vi "FPGA_FTL_trigger_camera_synchro_laser_lines.vi"(3 "N Z positions":i32) -> ()   [LabVIEW 2015]
uses:
  <vilib>/Platform/TimedLoop/XDataNode/timing_clust.ctl
  <vilib>/Platform/TimedLoop/XDataNode/nitl_modes.ctl
  <vilib>/Platform/TimedLoop/XDataNode/wakeup.ctl
  <vilib>/rvi/FXPMathLib/basic elements/FxpIntAccumulator/subVIs/nifxpmath_IntAccumulator_SimConfig.ctl
  <vilib>/rvi/Emulation/niFpgaGetClockAttributes.vi
  <vilib>/rvi/Emulation/niFpgaSctlEmulationGetInTimedLoop.vi
  <vilib>/rvi/Emulation/niFpgaEmulationReportErrorSimple.vi
  <vilib>/rvi/eio/common/nirviEmuTemplateMethod_errors.vi
  <vilib>/rvi/Emulation/niFpgaCriticalErrorInLSC.vi
  <vilib>/rvi/Emulation/niFpgaProcessEmulError.vi
  <vilib>/rvi/Analysis/common/codeGenErrors/XNode/niFpgaXNodeCodeGenErrorHandle.vi
  <vilib>/rvi/FXPMathLib/basic elements/FxpIntAccumulator/simVIs/DllFxpIntAccumulator_sub.vi
  <vilib>/eio/EIONode/EIONode.xnode
  <vilib>/rvi/Analysis/measure/dc-rms/XNode/niFpgaDC-RMS.xnode
  <vilib>/Platform/TimedLoop/XDataNode/XDataNode.xnode
  <vilib>/rvi/FXPMathLib/basic elements/FxpIntAccumulator/XNode/nifxpmath_IntAccumulator.xnode
  <vilib>/Platform/TimedLoop/XDataNode/XDNodeRunTimeDep.lvlib
panel:
  in  "stop":bool
  out "duration (ms)":u32
  out "QPD":T1
  in  "Reset counter":bool
  in  "Count(uSec)":u32=100
  out "Images acquired":i32
  in  "Laser lines":i32[](array[numeric])=[0, 0, 0, 0, 0]
  in  "Laser power":sgl[](array[numeric])=[0.0, 0.0, 0.0, 0.0, 0.0]
  in  "N laser lines":i32
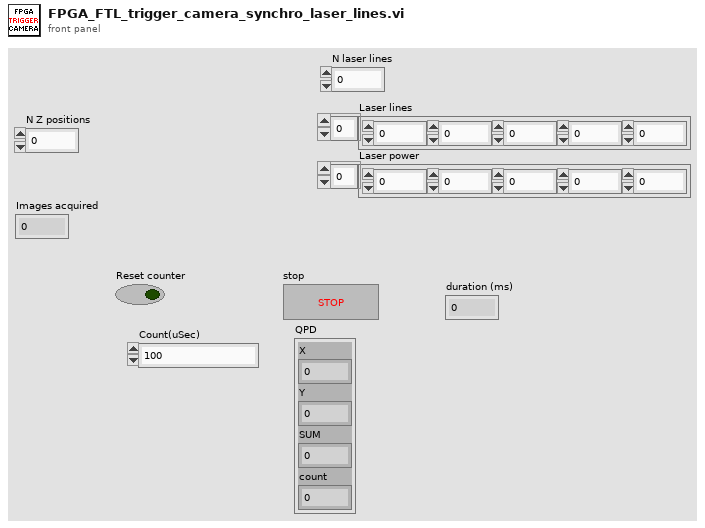
[diagram p1: front panel]
types:
  T1 = cluster{"X":sgl, "Y":sgl, "SUM":sgl, "count":u32}
  T2 = typedef "XDNodeRunTimeDep.lvlib/timing_clust.ctl" = cluster{"Expected End [f-1]":u64, "Actual End [f-1]":u64, "Finished Late? [f-1]":bool, "Expected End [i-1]":u64, "Actual End [i-1]":u64, "Finished Late? [i-1]":bool, "Expected Start [i]":u64, "Actual Start [i]":u64, "Expected Start [f]":u64, "Actual Start [f]":u64, "Source Name":string, "Structure Name":string, "Period":i64, "Deadline":i64, "Offset":i64, "Start":i64, "Priority":i32, "Timeout":i32, "Mode":T3, "Wakeup Reason":T4, "Error":errorcluster, "Source Type":string, "Secondary Source Type":string, "Global End Time":u64, "Global Start Time":u64, "Frame Duration":u64, "Iteration Duration":u64, "Assigned CPU":i32, "I/O Scan Engine Mode":u32}
  T3 = typedef "XDNodeRunTimeDep.lvlib/nitl_modes.ctl" = enum32{"No Change", "Process missed periods, maintain original phase", "Discard missed periods, maintain original phase", "Process missed periods, ignore original phase", "Discard missed periods, ignore original phase"}
  T4 = typedef "XDNodeRunTimeDep.lvlib/wakeup.ctl" = enum32{"Normal", "Aborted", "Asynchronous wakeup", "Timing source error", "Timed loop error", "Timeout"}
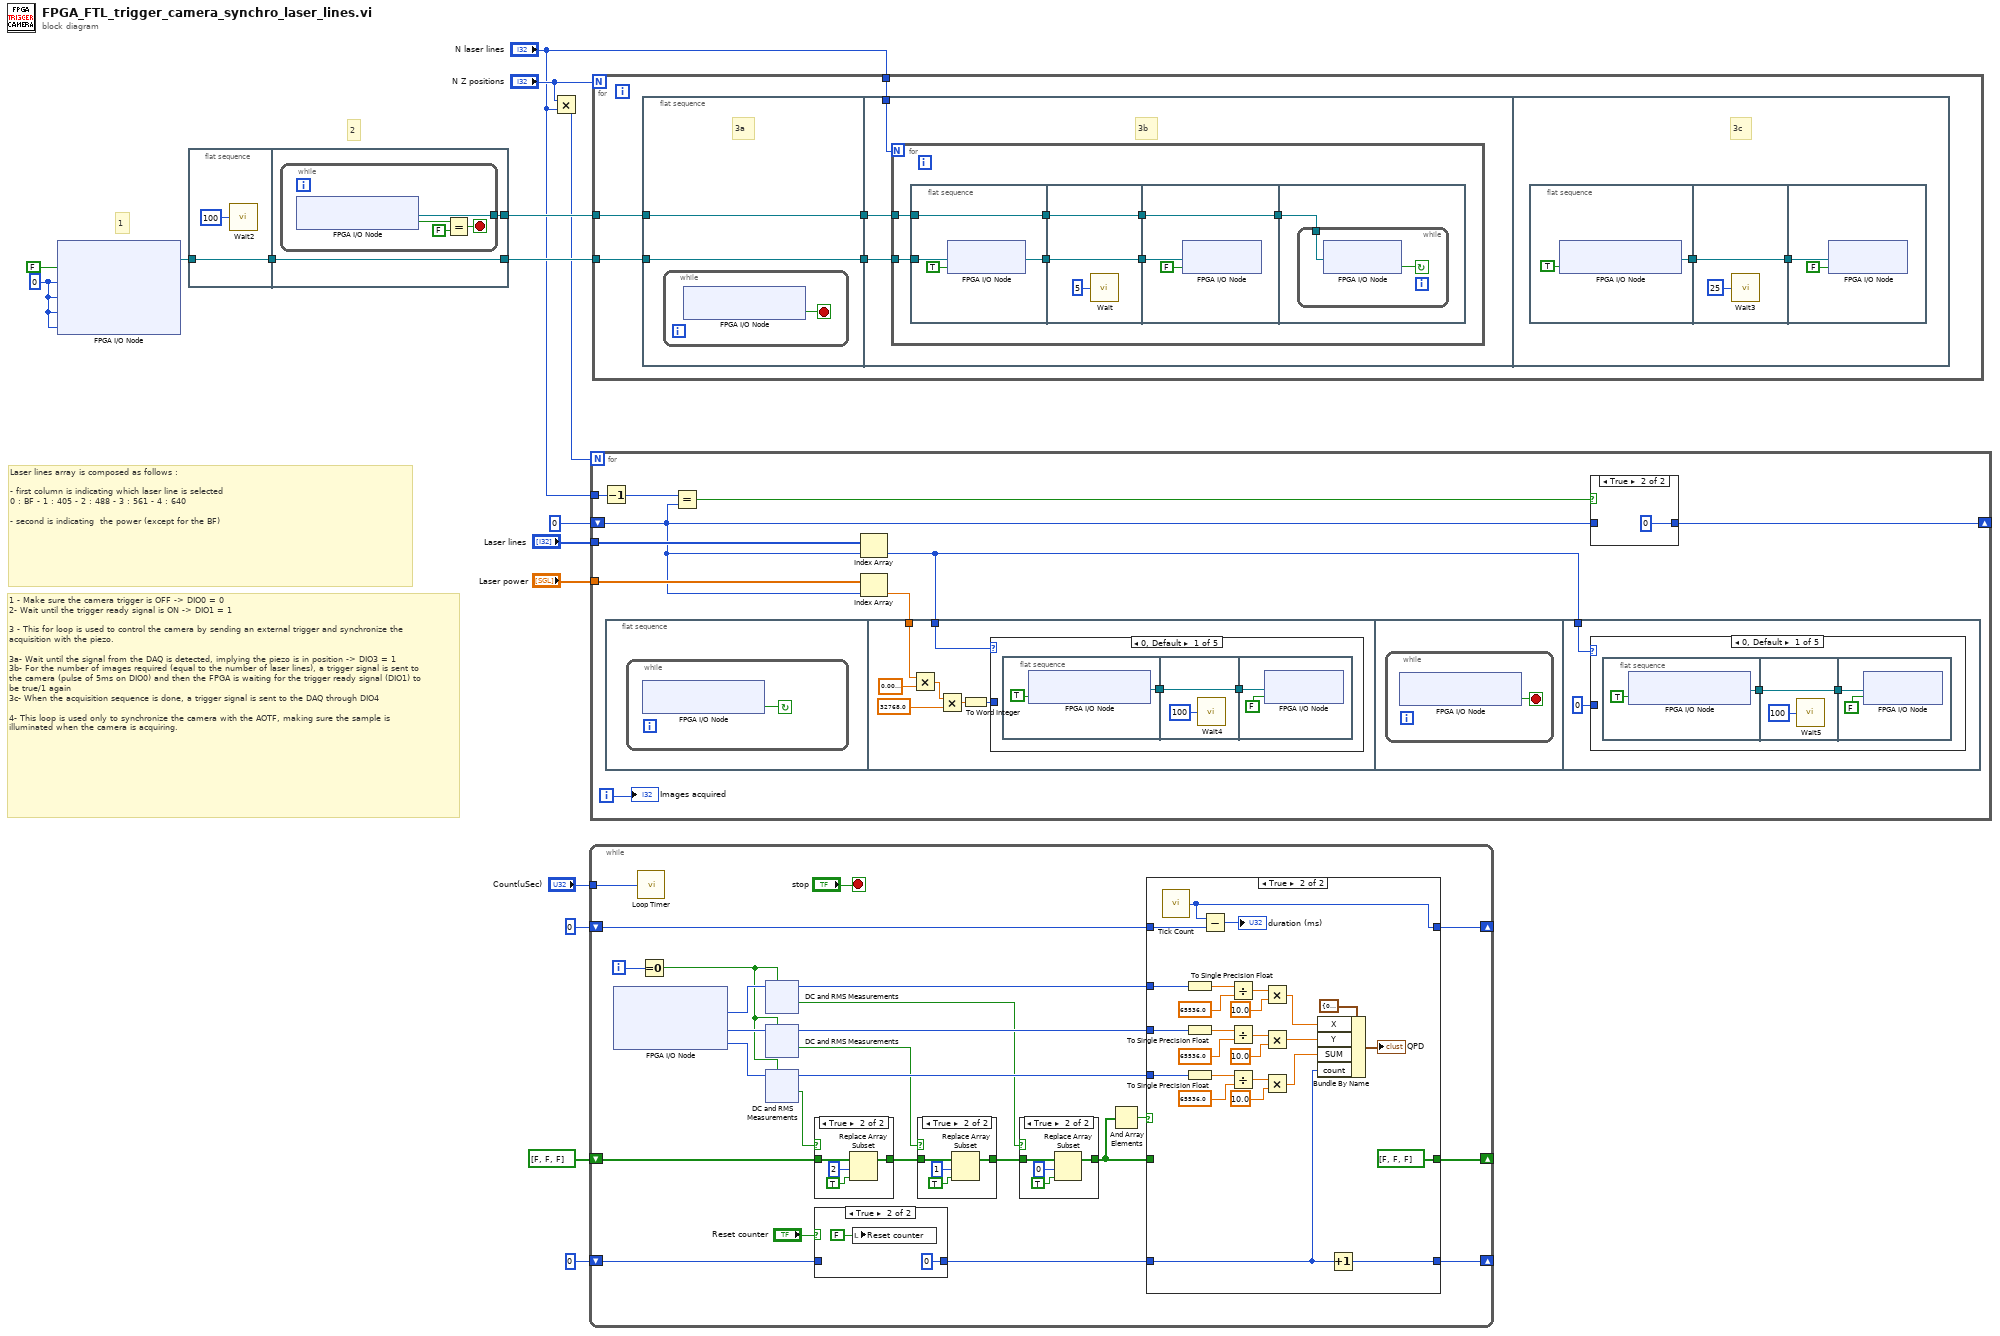
[diagram p0: block diagram]
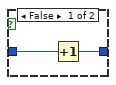
[diagram p7: hidden frame]
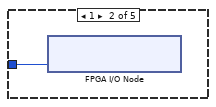
[diagram p8: hidden frame]
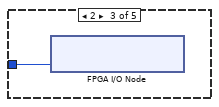
[diagram p9: hidden frame]
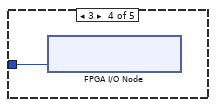
[diagram p10: hidden frame]
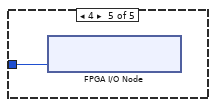
[diagram p11: hidden frame]
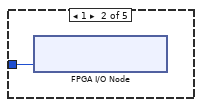
[diagram p12: hidden frame]
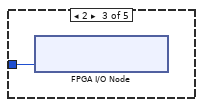
[diagram p13: hidden frame]
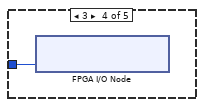
[diagram p14: hidden frame]
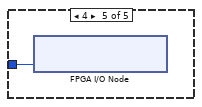
[diagram p15: hidden frame]
diagram:
  w5 = i16 0 ("Connector0/AO0")
  # "2"
  # "1"
  # "1 - Make sure the camera trigger is OFF -> DIO0 = 0\n2- Wait until the trigger ready signal is ON -> DIO1 = 1\n\n3 - This for loop is used to control the camera by sending an external trigger and synchronize the acquisition with the piezo.\n\n3a- Wait until the signal from the DAQ is detected, implying the piezo is in position -> DIO3 = 1 \n3b- For the number of images required (equal to the number of laser lines), a trigger signal is sent to the camera (pulse of 5ms on DIO0) and then the FPGA is waiting for the trigger ready signal (DIO1) to be true/1 again\n3c- When the acquisition sequence is done, a trigger signal is sent to the DAQ through DIO4\n\n4- This loop is used only to synchronize the camera with the AOTF, making sure the sample is illuminated when the camera is acquiring."
  # "Laser lines array is composed as follows :\n\n- first column is indicating which laser line is selected \n0 : BF - 1 : 405 - 2 : 488 - 3 : 561 - 4 : 640\n\n- second is indicating  the power (except for the BF)"
  n1 = xnode "FPGA I/O Node"("Connector0/DIO0"=FALSE, "Connector0/AO0"=w5, "Connector0/AO1"=w5, "Connector0/AO2"=w5, "Connector0/AO3"=w5) -> ("FPGA I/O Out"=w15:refnum<k21>)  [unwired: 5 in, 4 out]
  n2 = flat-sequence {
    tunnel: w15 -> [w18]
    tunnel: [w18] -> w14
    tunnel: w14 -> [w20]
    tunnel: [w20] -> w13
    tunnel: [w19] -> w12
    frame #0 {
      n3 = call "Wait2"("Count(uSec)"=u32 100 ("Count(mSec)")) -> ()  [unwired: 1 out]
    }
    frame #1 {
      n4 = while {
        tunnel: [w24] -> w19
        stop <- w21 stop-if-true
        n5 = xnode "FPGA I/O Node"() -> ("Connector0/DIO1"=w23:bool, "FPGA I/O Out"=w24:refnum<k21>)  [unwired: 1 in]
        n6 = Equal?(x=w23, y=FALSE) -> (x = y?=w21:bool)
      }
    }
  }
  n7 = Multiply(x="N Z positions", y="N laser lines") -> (x*y=w7:i32)
  n8 = while {
    shift-right: [w32] -> _
    shift-left: bool[] [FALSE, FALSE, FALSE] ("initialized array") -> [w40]
    shift-right: [w30] -> _
    shift-left: u32 0 -> [w31]
    tunnel: "Count(uSec)" -> [w29]
    shift-right: [w28] -> _
    shift-left: u32 0 -> [w26]
    i -> [w47]
    stop <- "stop" stop-if-true
    n9 = xnode "FPGA I/O Node"() -> ("Connector0/AI0"=w49:i16, "Connector0/AI1"=w45:i16, "Connector0/AI2"=w44:i16)  [unwired: 3 in, 3 out]
    n10 = call "Loop Timer"("Count(uSec)"=w29) -> ()  [unwired: 1 out]
    n11 = Equal To 0?(x=w47) -> (x = 0?=w41:bool)
    n12 = xnode "DC and RMS Measurements"("input data"=w49, "reset"=w41) -> ("DC"=w46:i16, "output valid"=w35:bool)
    n13 = xnode "DC and RMS Measurements"("input data"=w45, "reset"=w41) -> ("DC"=w43:i16, "output valid"=w36:bool)
    n14 = xnode "DC and RMS Measurements"("input data"=w44, "reset"=w41) -> ("DC"=w42:i16, "output valid"=w37:bool)
    n15 = case shown="True" w37 {
      tunnel: w40 -> [w58 w61]
      tunnel: [w58 w59] -> w39
      frame False {
      }
      frame True {
        n16 = Replace Array Subset(array=w61, new element=TRUE, index=2) -> (w59:bool[])
      }
    }
    n17 = case shown="True" "Reset counter" {
      tunnel: w26 -> [w50 _]
      tunnel: [w50 u32 0] -> w25
      frame False {
      }
      frame True {
        n18 = local write "Reset counter"(FALSE ("Reset counter")) -> ()
      }
    }
    n19 = case shown="True" w36 {
      tunnel: w39 -> [w63 w66]
      tunnel: [w63 w64] -> w38
      frame False {
      }
      frame True {
        n20 = Replace Array Subset(array=w66, new element=TRUE, index=1) -> (w64:bool[])
      }
    }
    n21 = case shown="True" w35 {
      tunnel: [w53 w55] -> w33
      tunnel: w38 -> [w53 w54]
      frame False {
      }
      frame True {
        n22 = Replace Array Subset(array=w54, new element=TRUE, index=0) -> (w55:bool[])
      }
    }
    n23 = And Array Elements(Boolean array=w33) -> (logical AND=w34:bool)
    n24 = case shown="True" w34 {
      tunnel: w46 -> [_ w96]
      tunnel: w43 -> [_ w87]
      tunnel: w42 -> [_ w82]
      tunnel: w33 -> [w70 _]
      tunnel: [w70 bool[] [FALSE, FALSE, FALSE] ("initialized array")] -> w32
      tunnel: w31 -> [w69 w77]
      tunnel: [w69 w75] -> w30
      tunnel: w25 -> [w68 w72]
      tunnel: [w68 w71] -> w28
      frame False {
      }
      frame True {
        n25 = call "Tick Count"() -> ("Tick Count(mSec)"=w75:u32)
        n26 = To Single Precision Float(number=w96) -> (single precision float=w95:sgl)
        n27 = To Single Precision Float(number=w87) -> (single precision float=w88:sgl)
        n28 = To Single Precision Float(number=w82) -> (single precision float=w86:sgl)
        n29 = Subtract(x=w75, y=w77) -> (x-y=→"duration (ms)":u32)
        n30 = Divide(x=w95, y=sgl 65536.0) -> (x/y=w93:sgl)
        n31 = Divide(x=w88, y=sgl 65536.0) -> (x/y=w90:sgl)
        n32 = Divide(x=w86, y=sgl 65536.0) -> (x/y=w84:sgl)
        n33 = Multiply(x=w93, y=sgl 10.0) -> (x*y=w81:sgl)
        n34 = Multiply(x=w90, y=sgl 10.0) -> (x*y=w80:sgl)
        n35 = Multiply(x=w84, y=sgl 10.0) -> (x*y=w79:sgl)
        n36 = Bundle By Name(cluster=T1 {"X"=0.0, "Y"=0.0, "SUM"=0.0, "count"=0} ("output cluster"), "X"=w81, "Y"=w80, "SUM"=w79, "count"=w72) -> (→"QPD":T1)
        n37 = Increment(x=w72) -> (x+1=w71:u32)
      }
    }
  }
  n38 = for {
    N: w7 -> [_]
    shift-right: [w359] -> _
    shift-left: 0 -> [w356]
    tunnel: "Laser lines" -> [w358]
    tunnel: "Laser power" -> [w357]
    tunnel: "N laser lines" -> [w354]
    i -> [w352]
    n39 = Decrement(x=w354) -> (x-1=w353:i32)
    n40 = flat-sequence {
      tunnel: w361 -> [w366]
      tunnel: w355 -> [w368]
      tunnel: w361 -> [w386]
      frame #0 {
        n41 = while {
          stop <- w365 continue-if-true
          n42 = xnode "FPGA I/O Node"() -> ("Connector0/DIO2"=w365:bool)  [unwired: 1 in, 1 out]
        }
      }
      frame #1 {
        n43 = Multiply(x=w368, y=sgl 0.01) -> (x*y=w367:sgl)
        n44 = Multiply(x=w367, y=sgl 32768.0) -> (x*y=w370:sgl)
        n45 = To Word Integer(number=w370) -> (16bit integer=w369:i16)
        n46 = case shown="0, Default" w366 {
          tunnel: w369 -> [_ w381 w382 w383 w384]
          frame 0, Default {
            n47 = flat-sequence {
              tunnel: [w375] -> w374
              tunnel: w374 -> [w377]
              tunnel: [w377] -> w373
              tunnel: w373 -> [w380]
              frame #0 {
                n48 = xnode "FPGA I/O Node"("Connector0/DIO5"=TRUE) -> ("FPGA I/O Out"=w375:refnum<k21>)  [unwired: 1 in]
              }
              frame #1 {
                n49 = call "Wait4"("Count(uSec)"=u32 100) -> ()  [unwired: 1 out]
              }
              frame #2 {
                n50 = xnode "FPGA I/O Node"("I/O Item"=FALSE, "FPGA I/O In"=w380) -> ()  [unwired: 1 out]
              }
            }
          }
          frame 1 {
            n51 = xnode "FPGA I/O Node"("Connector0/AO2"=w381) -> ()  [unwired: 1 in, 1 out]
          }
          frame 2 {
            n52 = xnode "FPGA I/O Node"("Connector0/AO3"=w382) -> ()  [unwired: 1 in, 1 out]
          }
          frame 3 {
            n53 = xnode "FPGA I/O Node"("Connector0/AO0"=w383) -> ()  [unwired: 1 in, 1 out]
          }
          frame 4 {
            n54 = xnode "FPGA I/O Node"("Connector0/AO1"=w384) -> ()  [unwired: 1 in, 1 out]
          }
        }
      }
      frame #2 {
        n55 = while {
          stop <- w385 stop-if-true
          n56 = xnode "FPGA I/O Node"() -> ("Connector0/DIO2"=w385:bool)  [unwired: 1 in, 1 out]
        }
      }
      frame #3 {
        n57 = case shown="0, Default" w386 {
          tunnel: i16 0 -> [_ w396 w397 w398 w399]
          frame 0, Default {
            n58 = flat-sequence {
              tunnel: [w390] -> w389
              tunnel: w389 -> [w392]
              tunnel: [w392] -> w388
              tunnel: w388 -> [w395]
              frame #0 {
                n59 = xnode "FPGA I/O Node"("Connector0/DIO5"=TRUE) -> ("FPGA I/O Out"=w390:refnum<k21>)  [unwired: 1 in]
              }
              frame #1 {
                n60 = call "Wait5"("Count(uSec)"=u32 100) -> ()  [unwired: 1 out]
              }
              frame #2 {
                n61 = xnode "FPGA I/O Node"("I/O Item"=FALSE, "FPGA I/O In"=w395) -> ()  [unwired: 1 out]
              }
            }
          }
          frame 1 {
            n62 = xnode "FPGA I/O Node"("Connector0/AO2"=w396) -> ()  [unwired: 1 in, 1 out]
          }
          frame 2 {
            n63 = xnode "FPGA I/O Node"("Connector0/AO3"=w397) -> ()  [unwired: 1 in, 1 out]
          }
          frame 3 {
            n64 = xnode "FPGA I/O Node"("Connector0/AO0"=w398) -> ()  [unwired: 1 in, 1 out]
          }
          frame 4 {
            n65 = xnode "FPGA I/O Node"("Connector0/AO1"=w399) -> ()  [unwired: 1 in, 1 out]
          }
        }
      }
    }
    n66 = Equal?(x=w353, y=w356) -> (x = y?=w360:bool)
    n67 = Index Array(array=w358, index=w356) -> (element=w361:i32)
    n68 = Index Array(array=w357, index=w356) -> (element=w355:sgl)
    n69 = case shown="True" w360 {
      tunnel: w356 -> [w363 _]
      tunnel: [w362 0] -> w359
      frame False {
        n70 = Increment(x=w363) -> (x+1=w362:i32)
      }
      frame True {
      }
    }
    "Images acquired" <- w352
  }
  n71 = for {
    N: "N Z positions" -> [_]
    tunnel: w13 -> [w403]
    tunnel: w12 -> [w404]
    tunnel: "N laser lines" -> [w400]
    n72 = flat-sequence {
      tunnel: w403 -> [w405]
      tunnel: w404 -> [w406]
      tunnel: [w406] -> w402
      tunnel: [w405] -> w401
      tunnel: w402 -> [w410]
      tunnel: w401 -> [w409]
      tunnel: w400 -> [w408]
      frame #0 {
        # "3a"
        n73 = while {
          stop <- w407 stop-if-true
          n74 = xnode "FPGA I/O Node"() -> ("Connector0/DIO3"=w407:bool)  [unwired: 1 in, 1 out]
        }
      }
      frame #1 {
        # "3b"
        n75 = for {
          N: w408 -> [_]
          tunnel: w410 -> [w412]
          tunnel: w409 -> [w411]
          n76 = flat-sequence {
            tunnel: [w420] -> w417
            tunnel: [w418] -> w416
            tunnel: w411 -> [w419]
            tunnel: w412 -> [w418]
            tunnel: w417 -> [w423]
            tunnel: [w423] -> w415
            tunnel: [w422] -> w414
            tunnel: w416 -> [w422]
            tunnel: w415 -> [w426]
            tunnel: [w425] -> w413
            tunnel: w414 -> [w425]
            tunnel: w413 -> [w428]
            frame #0 {
              n77 = xnode "FPGA I/O Node"("I/O Item"=TRUE ("Connector0/DIO0"), "FPGA I/O In"=w419) -> ("FPGA I/O Out"=w420:refnum<k21>)
            }
            frame #1 {
              n78 = call "Wait"("Count(mSec)"=u32 5) -> ()  [unwired: 1 out]
            }
            frame #2 {
              n79 = xnode "FPGA I/O Node"("I/O Item"=FALSE ("Connector0/DIO0"), "FPGA I/O In"=w426) -> ()  [unwired: 1 out]
            }
            frame #3 {
              n80 = while {
                tunnel: w428 -> [w430]
                stop <- w429 continue-if-true
                n81 = xnode "FPGA I/O Node"("FPGA I/O In"=w430) -> ("I/O Item"=w429:bool)  [unwired: 1 out]
              }
            }
          }
        }
      }
      frame #2 {
        # "3c"
        n82 = flat-sequence {
          tunnel: [w434] -> w432
          tunnel: w432 -> [w435]
          tunnel: [w435] -> w431
          tunnel: w431 -> [w437]
          frame #0 {
            n83 = xnode "FPGA I/O Node"("Connector0/DIO4"=TRUE) -> ("FPGA I/O Out"=w434:refnum<k21>)  [unwired: 1 in]
          }
          frame #1 {
            n84 = call "Wait3"("Count(mSec)"=u32 25) -> ()  [unwired: 1 out]
          }
          frame #2 {
            n85 = xnode "FPGA I/O Node"("I/O Item"=FALSE ("Connector0/DIO0"), "FPGA I/O In"=w437) -> ()  [unwired: 1 out]
          }
        }
      }
    }
  }
